vi "Change Bit Value - Multi.vi"(8 "error in (no error)":errorcluster, 9 "States":u8[](array[ring]) items=["0", "1", "Z", "L", "H", "X", "T", "V"], 10 "Bits":T1[](array[typedef]) items=["SDA", "SCL"], 11 "I2C waveform info":T2) -> (0 "error out":errorcluster, 3 "I2C waveform info out":T2)   [LabVIEW 2009, in "IDW.lvlib"]
doc: "Appends a single sample to the I2C waveform wherein both of the bus lines (SCL and SDA) change value."
uses:
  IDW.lvlib
  _Typedefs/Waveform info.ctl
  _Typedefs/Timing - ticks.ctl
  _Typedefs/Default transition action.ctl
  _Typedefs/Bit type.ctl
  _Typedefs/Channel Ring.ctl
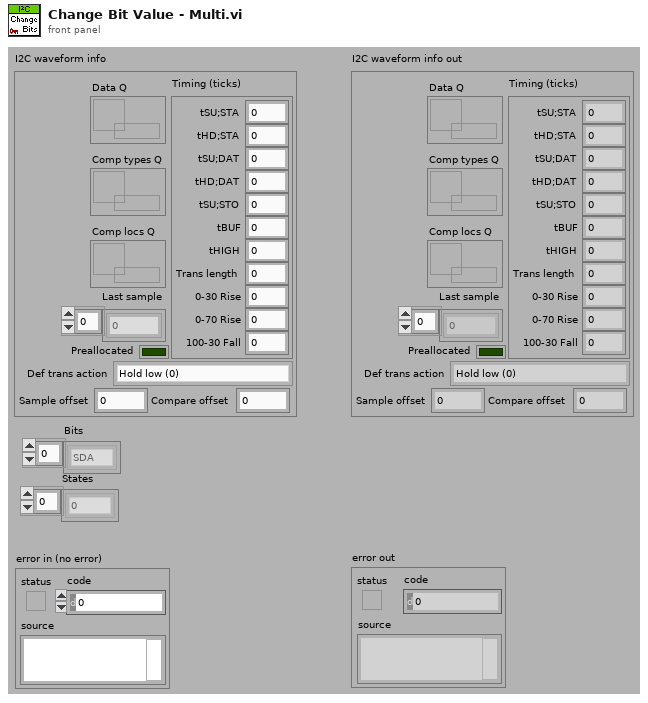
[diagram p1: front panel]
types:
  T1 = typedef "IDW.lvlib/Channel Ring.ctl" = u16
  T2 = typedef "IDW.lvlib/Waveform info.ctl" = cluster{"Last sample":u8[], "Sample offset":u64, "Compare offset":u64, "Timing (ticks)":T3, "Preallocated":bool, "Def trans action":T4, "Data Q":refnum<queue>, "Comp types Q":refnum<queue>, "Comp locs Q":refnum<queue>}
  T3 = typedef "IDW.lvlib/Timing - ticks.ctl" = cluster{"tSU;STA":i32, "tHD;STA":i32, "tSU;DAT":i32, "tHD;DAT":i32, "tSU;STO":i32, "tBUF":i32, "tHIGH":i32, "Trans length":i32, "0-30 Rise":i32, "0-70 Rise":i32, "100-30 Fall":i32}
  T4 = typedef "IDW.lvlib/Default transition action.ctl" = enum16{"Hold low (0)", "Release (Z)", "Set up next value", "Hold previous value", "Preserve tHD;DAT and tSU;DAT"}
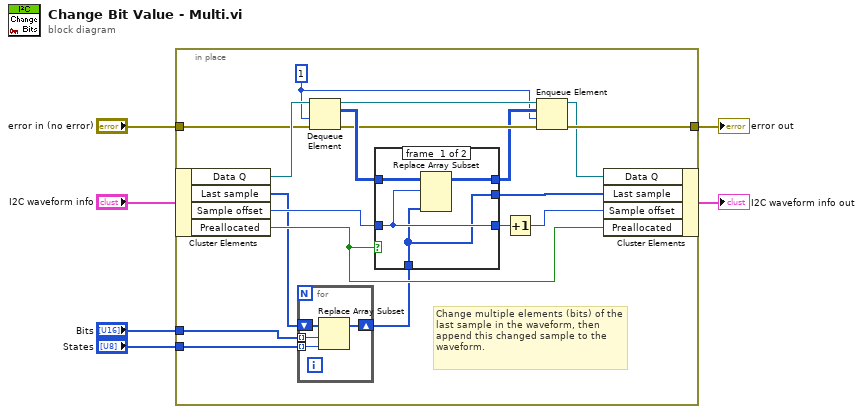
[diagram p0: block diagram]
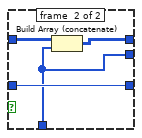
[diagram p2: hidden frame]
diagram:
  n1 = in-place {
    in-place-border: "Bits" -> [w18]
    in-place-border: "States" -> [w19]
    in-place-border: "error in (no error)" -> [w14]
    in-place-border: [w10] -> w1
    w7 = 1 ("timeout in ms (-1)")
    # "Change multiple elements (bits) of the last sample in the waveform, then append this changed sample to the waveform."
    n2 = in-place-cluster #1("I2C waveform info") -> ("Data Q"=w15:refnum<queue>, "Last sample"=w16:u8[], "Sample offset"=w22:u64, "Preallocated"=w23:bool)
    n3 = for {
      tunnel: w19 -> [w28] mode=indexing
      tunnel: w18 -> [w27] mode=indexing
      shift-right: [w26] -> w17
      shift-left: w16 -> [w25]
      n4 = Replace Array Subset(array=w25, new element=w28, index=w27) -> (w26:u8[])
    }
    n5 = Dequeue Element(queue=w15, timeout in ms (-1)=w7, error in (no error)=w14) -> (queue out=w12:refnum<queue>, element=w13:u8[][], error out=w11:errorcluster)  [unwired: 1 out]
    n6 = case shown="True" w23 {
      tunnel: w13 -> [w32 w36]
      tunnel: [w29 w33] -> w24
      tunnel: [w31 w35] -> w8
      tunnel: w22 -> [w30 w34]
      tunnel: [w30 w34] -> w21
      tunnel: w17 -> [w29 w33]
      frame #0 {
        n7 = Replace Array Subset(array=w32, new element=w29, index (row)=w30) -> (w31:u8[][])  [unwired: 1 in]
      }
      frame #1 {
        n8 = Build Array (concatenate)(w36, w33) -> (w35:u8[][])
      }
    }
    n9 = Increment(x=w21) -> (x+1=w20:u64)
    n10 = Enqueue Element(queue=w12, element=w8, timeout in ms (-1)=w7, error in (no error)=w11) -> (queue out=w9:refnum<queue>, error out=w10:errorcluster)  [unwired: 1 out]
    n11 = in-place-cluster #1("Data Q"=w9, "Last sample"=w24, "Sample offset"=w20, "Preallocated"=w23) -> (→"I2C waveform info out":T2)
  }
  "error out" <- w1
